vi "Wheel Set Value.vi"(10 "Shooter Wheel DevRef Out":T1={"Shooter Config reference"=refnum, "Shooter Data"={"MotorControlDevRef"={"DeviceStatus"={"status"=FALSE, "code"=0, "source"=""}, "Type"=enum."PWM", "PWM"={"PWM Channel"=enum."PWM 0", "DeadBand"={"Name"="", "maxPositivePwm"=0, "minPositivePwm"=0, "centerPwm"=0, "maxNegativePwm"=0, "minNegativePwm"=0, "angularRange"=0}}, "CAN"={"Device Number"=0, "SetOutput VI Ref"=variant(enum8{"Percent VBus", "Current", "Speed", "Position", "Voltage"} enum."Percent VBus"), "GetOutput VI Ref"=variant(refnum<k1> refnum), "Enable VI Ref"=variant(dbl 0.0), "Disable VI Ref"=variant(enum8{"Percent VBus", "Speed", "Position", "Slave", "Unchanged / Invalid", "Voltage Compensation", "Current", "Motion Profile"} enum."Percent VBus"), "Data"=variant}, "Invert"=FALSE}, "Set Point"=refnum, "Actual"=refnum}}, 11 "RPM Desired":dbl) -> ()   [LabVIEW 2016, in "Wheel.lvlib"]
doc: "Help by FRC Team 836 - The RoboBees\n\nThis VI sets the Revolutions Per Minute (RPM) of a wheel."
uses:
  <userlib>/836-Library/Motion_Control/Shooter_Wheel/Wheel.lvlib
  <vilib>/Rock Robotics/SystemInterfaces/DIO/FPGA_DIOPWMChannel.ctl
  <vilib>/Rock Robotics/WPI/PWM/WPI_PWMDeadband.ctl
  <vilib>/Rock Robotics/WPI/MotorControl/WPI_MotorControlDeviceRef.ctl
  <userlib>/836-Libraries/Motion_Control/Shooter_Wheel/Data.ctl
  <userlib>/836-Libraries/Motion_Control/Shooter_Wheel/Config.ctl
  <userlib>/836-Libraries/Motion_Control/Shooter_Wheel/WheelControl.ctl
  <vilib>/Rock Robotics/WPI/MotorControl/WPI_MotorControlType.ctl
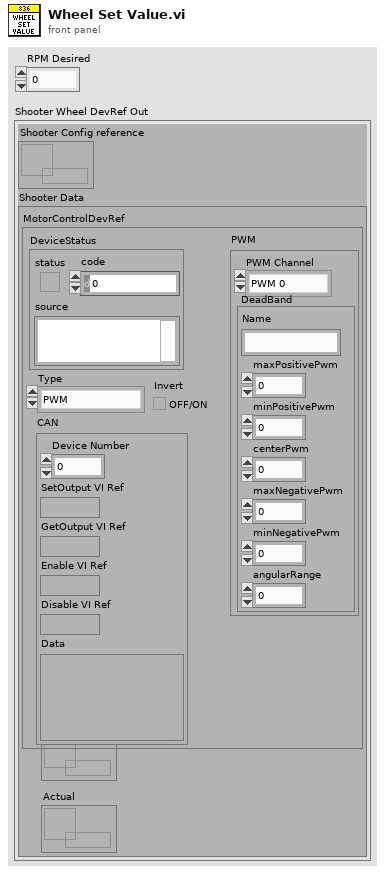
[diagram p1: front panel]
types:
  T1 = typedef "Wheel.lvlib/WheelControl.ctl" = cluster{"Shooter Config reference":refnum<data-value>, "Shooter Data":T2}
  T2 = typedef "Wheel.lvlib/Data.ctl" = cluster{"MotorControlDevRef":T3, "Set Point":refnum<k33>, "Actual":refnum<k33>}
  T3 = typedef "WPI_MotorControlDeviceRef.ctl" = cluster{"DeviceStatus":errorcluster, "Type":T4, "PWM":cluster{"PWM Channel":T5, "DeadBand":T6}, "CAN":cluster{"Device Number":u8, "SetOutput VI Ref":variant, "GetOutput VI Ref":variant, "Enable VI Ref":variant, "Disable VI Ref":variant, "Data":variant}, "Invert":bool}
  T4 = typedef "WPI_MotorControlType.ctl" = enum16{"PWM", "CAN"}
  T5 = typedef "FPGA_DIOPWMChannel.ctl" = enum8{"PWM 0", "PWM 1", "PWM 2", "PWM 3", "PWM 4", "PWM 5", "PWM 6", "PWM 7", "PWM 8", "PWM 9", "PWM MXP 0", "PWM MXP 1", "PWM MXP 2", "PWM MXP 3", "PWM MXP 4", "PWM MXP 5", "PWM MXP 6", "PWM MXP 7", "PWM MXP 8", "PWM MXP 9", "Invalid"}
  T6 = typedef "WPI_PWMDeadband.ctl" = cluster{"Name":string, "maxPositivePwm":i32, "minPositivePwm":i32, "centerPwm":i32, "maxNegativePwm":i32, "minNegativePwm":i32, "angularRange":u16}
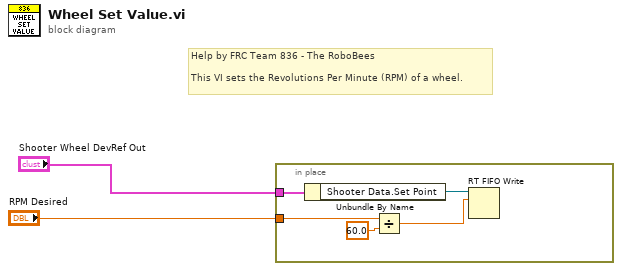
[diagram p0: block diagram]
diagram:
  # "Help by FRC Team 836 - The RoboBees\n\nThis VI sets the Revolutions Per Minute (RPM) of a wheel."
  n1 = in-place {
    in-place-border: "Shooter Wheel DevRef Out" -> [w7]
    in-place-border: "RPM Desired" -> [w5]
    n2 = Unbundle By Name(w7) -> ("Shooter Data.Set Point"=w6:refnum<k33>)
    n3 = Divide(x=w5, y=60.0) -> (x/y=w4:dbl)
    n4 = RT FIFO Write(0:w6, 1:w4) -> ()  [unwired: 3 in, 4 out]
  }
